vi "Parse Face Line From OBJ.vi"(11 "Face string":string) -> (1 "Normal Index":cluster{"x":i32, "y":i32, "z":i32}, 2 "Texture Index":cluster{"x":i32, "y":i32, "z":i32}, 3 "Vertex Index":cluster{"x":i32, "y":i32, "z":i32})   [LabVIEW 2020, in "3D.lvlib"]
uses:
  3D.lvlib
  <userlib>/_OpenG.lib/string/string.llb/openg_string.lvlib
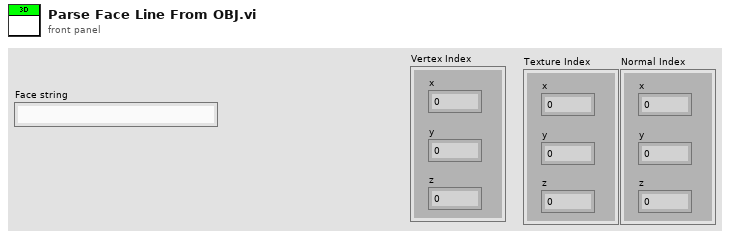
[diagram p1: front panel]
types:
  T1 = cluster{"default value 1":i32, "default value 1":i32, "default value 1":i32}
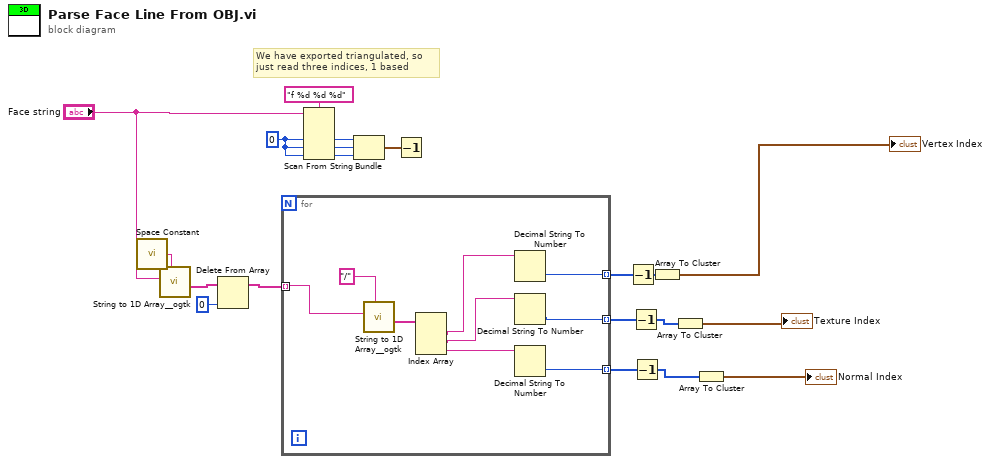
[diagram p0: block diagram]
diagram:
  w16 = 0 ("default value 1")
  # "We have exported triangulated, so just read three indices, 1 based"
  n1 = call <vilib>:"Space Constant.vi"() -> ("String"=w13:string)
  n2 = call <userlib>:"String to 1D Array__ogtk.vi"("delimiter (Tab)"=w13, "string"="Face string") -> ("Array of Strings"=w12:string[])  [unwired: 9 in]
  n3 = Delete From Array(array=w12, index=0) -> (array with subset deleted=w11:string[])  [unwired: 1 in, 1 out]
  n4 = for {
    tunnel: w11 -> [w29] mode=indexing
    tunnel: [w23] -> w8 mode=indexing
    tunnel: [w22] -> w7 mode=indexing
    tunnel: [w21] -> w9 mode=indexing
    n5 = call <userlib>:"String to 1D Array__ogtk.vi"("delimiter (Tab)"="/", "string"=w29) -> ("Array of Strings"=w27:string[])  [unwired: 9 in]
    n6 = Index Array(array=w27) -> (element #1=w26:string, element #2=w25:string, element #3=w24:string)  [unwired: 3 in]
    n7 = Decimal String To Number(string=w26) -> (number=w23:i32)  [unwired: 2 in, 1 out]
    n8 = Decimal String To Number(string=w25) -> (number=w22:i32)  [unwired: 2 in, 1 out]
    n9 = Decimal String To Number(string=w24) -> (number=w21:i32)  [unwired: 2 in, 1 out]
  }
  n10 = Scan From String(format string="f %d %d %d", input string="Face string", default 1=w16, default 2=w16, default 3=w16) -> (output 1=w17:i32, output 2=w18:i32, output 3=w19:i32)  [unwired: 2 in, 3 out]
  n11 = Bundle("default value 1"=w17, "default value 1"=w18, "default value 1"=w19) -> (w20:T1)  [unwired: 1 in]
  n12 = Decrement(x=w20) -> ()  [unwired: 1 out]
  n13 = Decrement(x=w8) -> (x-1=w6:i32[])
  n14 = Decrement(x=w7) -> (x-1=w4:i32[])
  n15 = Decrement(x=w9) -> (x-1=w2:i32[])
  n16 = Array To Cluster(array=w6) -> (cluster=→"Vertex Index":cluster{"[0]":i32, "[1]":i32, "[2]":i32})
  n17 = Array To Cluster(array=w4) -> (cluster=→"Texture Index":cluster{"[0]":i32, "[1]":i32, "[2]":i32})
  n18 = Array To Cluster(array=w2) -> (cluster=→"Normal Index":cluster{"[0]":i32, "[1]":i32, "[2]":i32})
